vi "Init from Ref.vi"(8 "error in":errorcluster, 10 "Font":refnum<k24>) -> (0 "error out":errorcluster, 3 "Font out":refnum<class "Font.lvclass">)   [LabVIEW 2023, in "SourceGrid.lvlib" / "Font.lvclass"]
uses:
  Font.lvclass
  System.Drawing
  Font.lvclass/Font.ctl
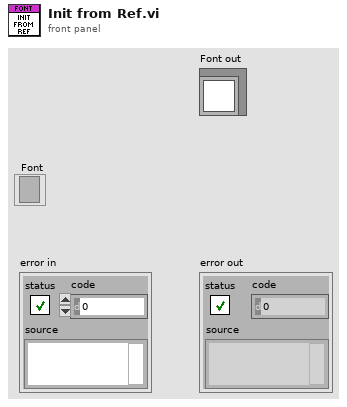
[diagram p1: front panel]
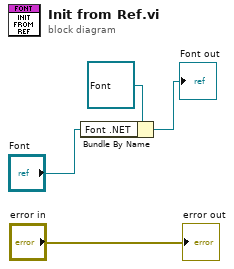
[diagram p0: block diagram]
diagram:
  n1 = Bundle By Name(cluster=refnum<class "Font.lvclass"> refnum ("SourceGrid.lvlib:Font.lvclass"), "Font .NET"="Font") -> (→"Font out":refnum<class "Font.lvclass">)
  "error out" <- "error in"
